vi "Boiler Start.vi"(8 "error in (no error)":errorcluster, 9 "Boiler Controls":T1 {"Fuel Valve Position" min=0.0 max=100.0 scale=0.0..100.0 scale format="%.2f"}, 10 "Indicator states in":T3 {"Time Count" format="%.2g"}, 11 "Runtime statuses in":T2) -> (0 "error out":errorcluster, 2 "Indicator states out":T3 {"Time Count" format="%.2g"}, 3 "Runtime statuses out":T2)   [LabVIEW 2014]
doc: "Checks runtime statuses. If pilot is proven and fuel valve is open more than 10% Boiler starts"
uses:
  Controls/Boiler Status Indicators.ctl
  Controls/Boiler runtime status indicators.ctl
  Controls/Boiler Controls.ctl
  Controls/Log file FGV action enum.ctl
  Controls/Log event enum.ctl
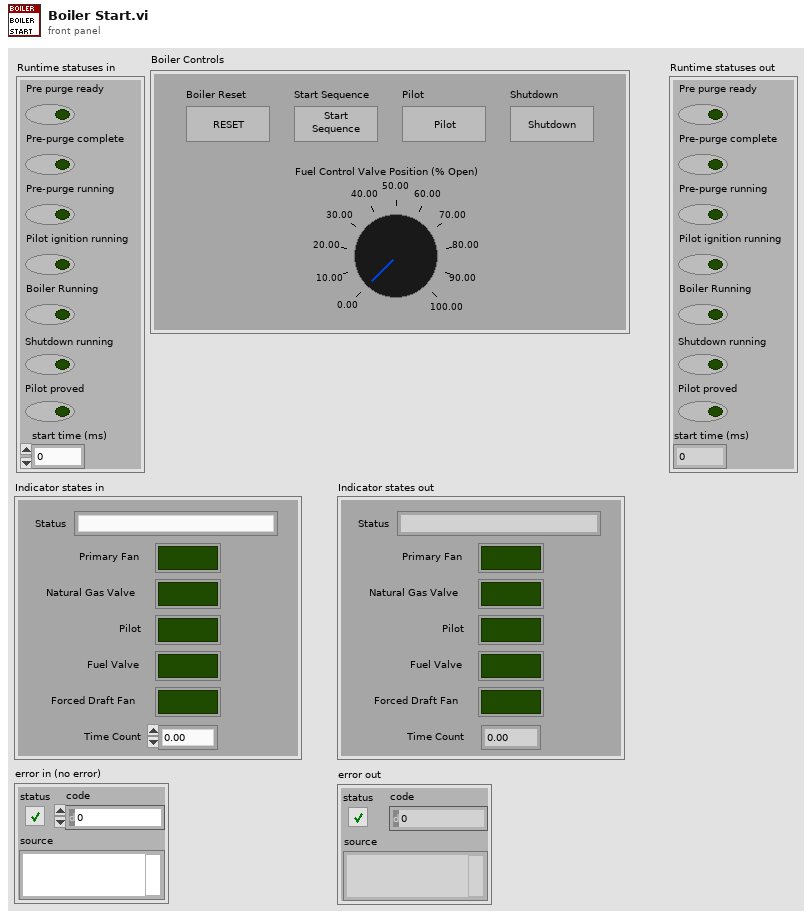
[diagram p1: front panel]
types:
  T1 = typedef "Boiler Controls.ctl" = cluster{"Boiler Reset":bool, "Start Sequence":bool, "Pilot":bool, "Shutdown":bool, "Fuel Valve Position":dbl}
  T2 = typedef "Boiler runtime status indicators.ctl" = cluster{"Pre purge ready":bool, "Pre-purge complete":bool, "Pre-purge running":bool, "Pilot ignition running":bool, "Boiler Running":bool, "Shutdown running":bool, "Pilot proved":bool, "start time (ms)":u32}
  T3 = typedef "Boiler Status Indicators.ctl" = cluster{"Status":string, "Primary Fan":bool, "Natural Gas Valve":bool, "Pilot":bool, "Fuel Valve":bool, "Forced Draft Fan":bool, "Time Count":dbl}
  T4 = typedef "Log event enum.ctl" = enum16{"Boiler Initialized", "Boiler Ready", "Start Pre-Purge", "Pre-Purge Complete", "Pilot ON", "Pilot proved", "Forced Draft Fan ON", "Boiler Running", "Start Shutdown Purge", "Shutdown Purge Complete"}
  T5 = typedef "Log file FGV action enum.ctl" = enum16{"open log file", "log event", "close log file"}
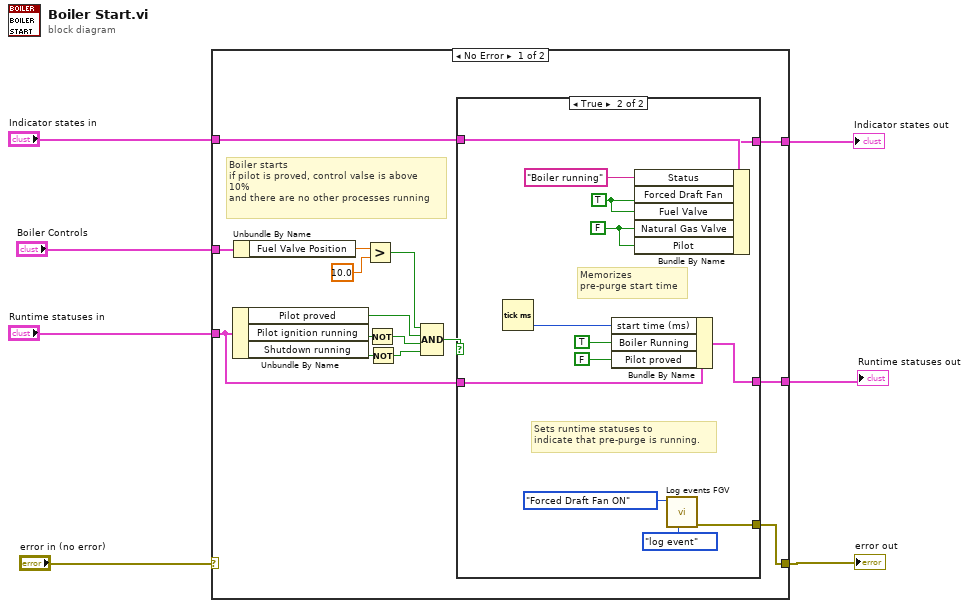
[diagram p0: block diagram]
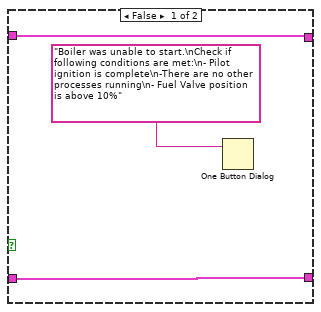
[diagram p2: hidden frame]
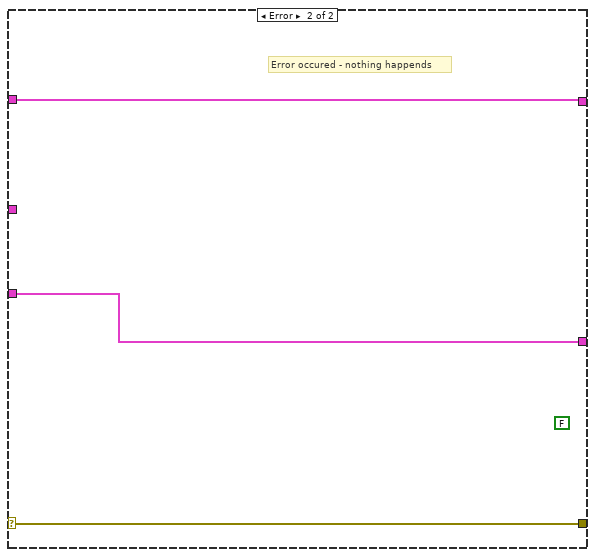
[diagram p3: hidden frame]
diagram:
  n1 = case shown="No Error" "error in (no error)" {
    selector: "error in (no error)" -> [_ w41]
    tunnel: [w8 w41] -> w6
    tunnel: "Runtime statuses in" -> [w15 w39]
    tunnel: "Indicator states in" -> [w17 w40]
    tunnel: [w16 w40] -> w3
    tunnel: [w14 w39] -> w2
    tunnel: "Boiler Controls" -> [w12 _]
    frame No Error {
      # "Boiler starts\nif pilot is proved, control valse is above\n10%\nand there are no other processes running"
      n2 = Unbundle By Name(w15) -> ("Pilot proved"=w13:bool, "Pilot ignition running"=w21:bool, "Shutdown running"=w22:bool)
      n3 = Unbundle By Name(w12) -> ("Fuel Valve Position"=w11:dbl)
      n4 = Greater?(x=w11, y=10.0) -> (0:w9:bool)
      n5 = Not(x=w21) -> (.not. x?=w20:bool)
      n6 = Not(x=w22) -> (.not. x?=w19:bool)
      n7 = Compound Arithmetic op=AND(w9, w13, w20, w19) -> (w18:bool)
      n8 = case shown="True" w18 {
        tunnel: w17 -> [w25 w38]
        tunnel: [w25 w37] -> w16
        tunnel: w15 -> [w24 w35]
        tunnel: [w24 w34] -> w14
        tunnel: [_ w26] -> w8
        frame False {
          n9 = One Button Dialog(message="Boiler was unable to start.\nCheck if following conditions are met:\n- Pilot ignition is complete\n-There are no other processes running\n- Fuel Valve position is above 10%") -> ()  [unwired: 1 in, 1 out]
        }
        frame True {
          w29 = FALSE ("Fuel Valve")
          w30 = TRUE ("Primary Fan")
          # "Memorizes\npre-purge start time"
          # "Sets runtime statuses to\nindicate that pre-purge is running."
          n10 = Tick Count (ms)() -> (millisecond timer value=w31:u32)
          n11 = Bundle By Name(cluster=w35, "start time (ms)"=w31, "Boiler Running"=TRUE ("Pre purge ready"), "Pilot proved"=FALSE ("Pre purge ready")) -> (w34:T2)
          n12 = Bundle By Name(cluster=w38, "Status"="Boiler running", "Forced Draft Fan"=w30, "Fuel Valve"=w30, "Natural Gas Valve"=w29, "Pilot"=w29) -> (w37:T3)
          n13 = call "Log events FGV.vi"("action"=Log_file_FGV_action_enum."log event", "Log event"=Log_event_enum."Forced Draft Fan ON") -> ("error out"=w26:errorcluster)  [unwired: 9 in]
        }
      }
    }
    frame Error {
      (unwired) FALSE
      # "Error occured - nothing happends"
    }
  }
  "Indicator states out" <- w3
  "error out" <- w6
  "Runtime statuses out" <- w2
